vi "Get All From Type Map.vi"(8 "error in (no error)":errorcluster, 11 "TwinCAT ADS in":refnum<class "TwinCAT ADS.lvclass">) -> (0 "error out":errorcluster, 2 "[.NET AdsDataType]":refnum<k24>[](array[refnum]), 3 "TwinCAT ADS out":refnum<class "TwinCAT ADS.lvclass">)   [LabVIEW 2018, in "TwinCAT ADS.lvclass"]
uses:
  TwinCAT ADS.lvclass
  TwinCAT.Ads
  TwinCAT ADS.lvclass/TwinCAT ADS.ctl
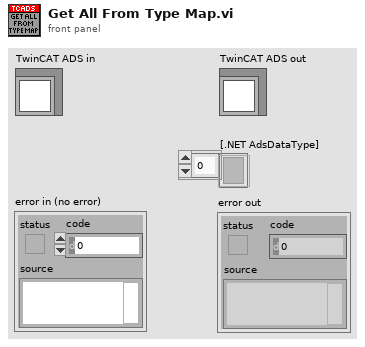
[diagram p1: front panel]
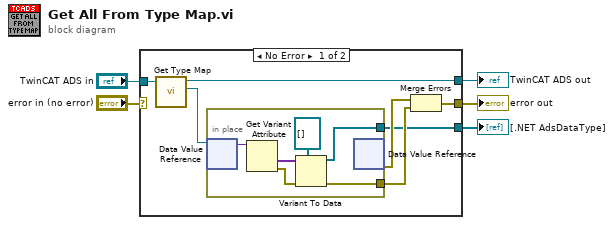
[diagram p0: block diagram]
diagram:
  n1 = case shown="No Error" "error in (no error)" {
    selector: "error in (no error)" -> [_ w19]
    tunnel: "TwinCAT ADS in" -> [w12 w20]
    tunnel: [w10 w20] -> w4
    tunnel: [w7 w19] -> w3
    tunnel: [w6 _] -> w1
    frame No Error {
      n2 = call "Get Type Map.vi"("TwinCAT ADS in"=w12) -> ("Type Map"=w11:refnum<data-value>, "TwinCAT ADS out"=w10:refnum<class "TwinCAT ADS.lvclass">)  [unwired: 8 in, 1 out]
      n3 = in-place {
        in-place-border: [w15] -> w6
        in-place-border: [w13] -> w8
        n4 = in-place-dvr #1(w11) -> (w18:variant)  [unwired: 1 out]
        n5 = Get Variant Attribute(Variant=w18) -> (values=w17:variant[], error out=w14:errorcluster)  [unwired: 3 in, 2 out]
        n6 = Variant To Data(error in=w14, type=refnum<k24>[] [], Variant=w17) -> (data=w15:refnum<k24>[], error out=w13:errorcluster)
        n7 = in-place-dvr #1() -> (w9:errorcluster)  [unwired: 1 in, 1 out]
      }
      n8 = Merge Errors(w9, w8) -> (w7:errorcluster)
    }
    frame Error {
    }
  }
  "error out" <- w3
  "TwinCAT ADS out" <- w4
  "[.NET AdsDataType]" <- w1
